vi "random_element.vi"(11 "Array In":dbl[](array[numeric])) -> (2 "Index":dbl, 3 "Random Element":dbl)   [LabVIEW 2016]
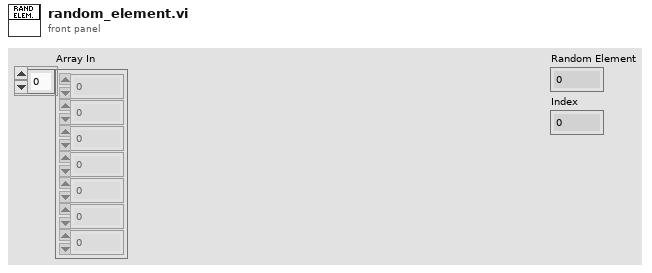
[diagram p1: front panel]
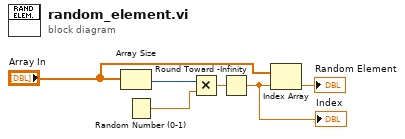
[diagram p0: block diagram]
diagram:
  n1 = Array Size(array="Array In") -> (size(s)=w5:i32)
  n2 = Random Number (0-1)() -> (number: 0 to 1=w6:dbl)
  n3 = Multiply(x=w5, y=w6) -> (x*y=w4:dbl)
  n4 = Round Toward -Infinity(1:w4) -> (0:w3:dbl)
  "Index" <- w3
  n5 = Index Array(array="Array In", index=w3) -> (element=→"Random Element":dbl)
